vi "Serializer Test Suite.vi"() -> ()   [LabVIEW 2013]
uses:
  <vilib>/addons/_JKI Toolkits/Caraya/classes/Test/Test.lvclass
panel:
  out "error out":errorcluster
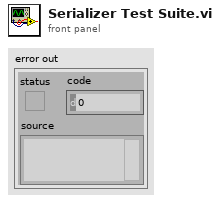
[diagram p1: front panel]
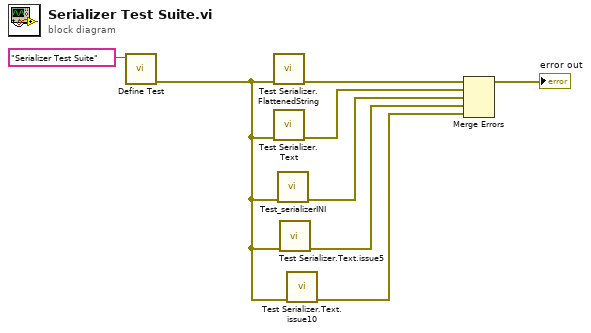
[diagram p0: block diagram]
diagram:
  n1 = call <vilib>:"Define Test.vi"("Label (VI Title)"="Serializer Test Suite") -> ("error out"=w2:errorcluster)  [unwired: 10 in]
  n2 = call "Test Serializer.FlattenedString.vi"("error in (no error)"=w2) -> ("error out"=w7:errorcluster)  [unwired: 10 in]
  n3 = call "Test Serializer.Text.vi"("error in (no error)"=w2) -> ("error out"=w5:errorcluster)  [unwired: 10 in]
  n4 = call "Test_serializerINI.vi"("error in (no error)"=w2) -> ("error out"=w4:errorcluster)  [unwired: 10 in]
  n5 = call "Test Serializer.Text.issue5.vi"("error in (no error)"=w2) -> ("error out"=w3:errorcluster)  [unwired: 10 in]
  n6 = call "Test Serializer.Text.issue10.vi"("error in (no error)"=w2) -> ("error out"=w1:errorcluster)  [unwired: 10 in]
  n7 = Merge Errors(w7, w5, w4, w3, w1) -> (→"error out":errorcluster)
